vi "Actor Core.vi"(8 "error in":errorcluster, 11 "EventHandlerTask in":refnum<class "EventHandlerTask.lvclass">) -> (0 "error out":errorcluster, 3 "Actor out":refnum<class "Actor.lvclass">)   [LabVIEW 2020, in "Volatus.lvlib" / "EventHandlerTask.lvclass"]
doc: "(<B>Filename</B>: Actor Framework.lvlib:Actor.lvclass:Actor Core.vi)\n\nReceives messages to the actor, reacts to them, and initiates any error handling that may shut the actor down.\n\nDescendant classes may override this VI to append parallel tasks for the actor to complete while it handles messages. Overrides use the Call Parent Class Method node."
uses:
  EventHandlerTask.lvclass
  EventHandlerTask.lvclass/EventHandlerTask.ctl
  <vilib>/ActorFramework/Actor/Actor.lvclass
  C:/Program Files (x86)/National Instruments/LabVIEW 2020/vi.lib/ActorFramework/Actor/Actor.lvclass
  C:/dev/lv20CE/relink/lv-volatus/Volatus/EventHandlerTask/EventHandlerTask.lvclass
  C:/dev/lv20CE/relink/lv-volatus/Volatus/EventHandler/EventHandler.lvclass
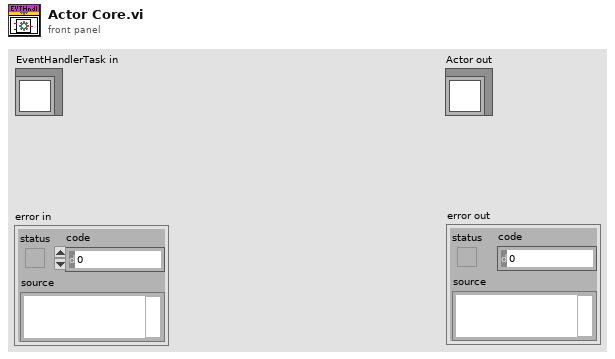
[diagram p1: front panel]
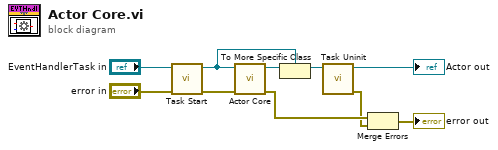
[diagram p0: block diagram]
diagram:
  n1 = call-dynamic "Task Start.vi"("error in (no error)"="error in", "EventHandlerTask in"="EventHandlerTask in") -> ("error out"=w3:errorcluster, "EventHandlerTask out"=w1:refnum<class "EventHandlerTask.lvclass">)  [unwired: 8 in]
  n2 = call-parent "Actor Core.vi"("error in"=w3, "Actor in"=w1) -> ("error out"=w9:errorcluster, "Actor out"=w8:refnum<class "Actor.lvclass">)  [unwired: 8 in]
  n3 = To More Specific Class(target class=w1, reference=w8) -> (specific class reference=w7:refnum<class "EventHandlerTask.lvclass">)  [unwired: 1 in, 1 out]
  n4 = call-dynamic "Task Uninit.vi"("EventHandlerTask in"=w7) -> ("error out"=w4:errorcluster, "EventHandlerTask out"=→"Actor out":refnum<class "EventHandlerTask.lvclass">)  [unwired: 9 in]
  n5 = Merge Errors(w9, w4) -> (→"error out":errorcluster)
